vi "DynamicPersonality.vi"(7 "Pinned":T1={"Attacker"="Auto", "Striker"="Auto", "Defender"="Auto"}, 10 "our_goalie_id":dbl, 11 "input cluster":T3={"our_robots"=[], "enemy_robots"=[], "balls"=[], "geometry"={"line_width"=0, "field_length"=0, "field_width"=0, "boundary_width"=0, "referee_width"=0, "goal_width"=0, "goal_depth"=0, "goal_wall_width"=0, "center_circle_radius"=0, "defense_radius"=0, "defense_stretch"=0, "free_kick_from_defense_dist"=0, "penalty_spot_from_field_line_dist"=0, "penalty_line_from_spot_dist"=0}, "IA Judge"={"stage"="", "command"="", "our_goalie_id"=0.0, "enemy_goalie_id"=0.0, "command\nenum"=enum."Halt", "Time"=enum."Azul"}, "Received Timestamp"=timestamp(0 s since 1904-01-01), "Events"={"Touch"=FALSE, "Ball out"=FALSE, "id touch"=0.0, "Ball out of \nVision"=FALSE, "Ball inside \nGoalie area"=FALSE, "Robot not responding"=FALSE, "Robots responding status"=[1.0, 1.0, 1.0, 1.0, 1.0, 1.0], "Enemy Ball \nPossession"=FALSE}}) -> (2 "output cluster":T3={"our_robots"=[], "enemy_robots"=[], "balls"=[], "geometry"={"line_width"=0, "field_length"=0, "field_width"=0, "boundary_width"=0, "referee_width"=0, "goal_width"=0, "goal_depth"=0, "goal_wall_width"=0, "center_circle_radius"=0, "defense_radius"=0, "defense_stretch"=0, "free_kick_from_defense_dist"=0, "penalty_spot_from_field_line_dist"=0, "penalty_line_from_spot_dist"=0}, "IA Judge"={"stage"="", "command"="", "our_goalie_id"=0.0, "enemy_goalie_id"=0.0, "command\nenum"=enum."Halt", "Time"=enum."Azul"}, "Received Timestamp"=timestamp(0 s since 1904-01-01), "Events"={"Touch"=FALSE, "Ball out"=FALSE, "id touch"=0.0, "Ball out of \nVision"=FALSE, "Ball inside \nGoalie area"=FALSE, "Robot not responding"=FALSE, "Robots responding status"=[1.0, 1.0, 1.0, 1.0, 1.0, 1.0], "Enemy Ball \nPossession"=FALSE}})   [LabVIEW 2016]
uses:
  Core/AI Input.ctl
  Core/AI Robot.ctl
  Intel/Functions Enum.ctl
  Intel/AttackerStates.ctl
  Core/AI Ball.ctl
  Core/Field Size.ctl
  Core/AI Judge.ctl
  Intel/Command Enum.ctl
  Select Personalitys.ctl
  Util/Select Auto None or Robot.ctl
panel:
  out "Dfdr\nPinned?":bool
  in  "Qtd Min p/ Stk":dbl=5.0
  out "Strk\nPinned?":bool
  out "Attck\nPinned?":bool
  in  "Ids validos":u32[](array[numeric])=[42, 42, 42, 42, 42, 42, 42]
  out "Maior prioridade de \natacante é o mais\nproximo da bola?":bool
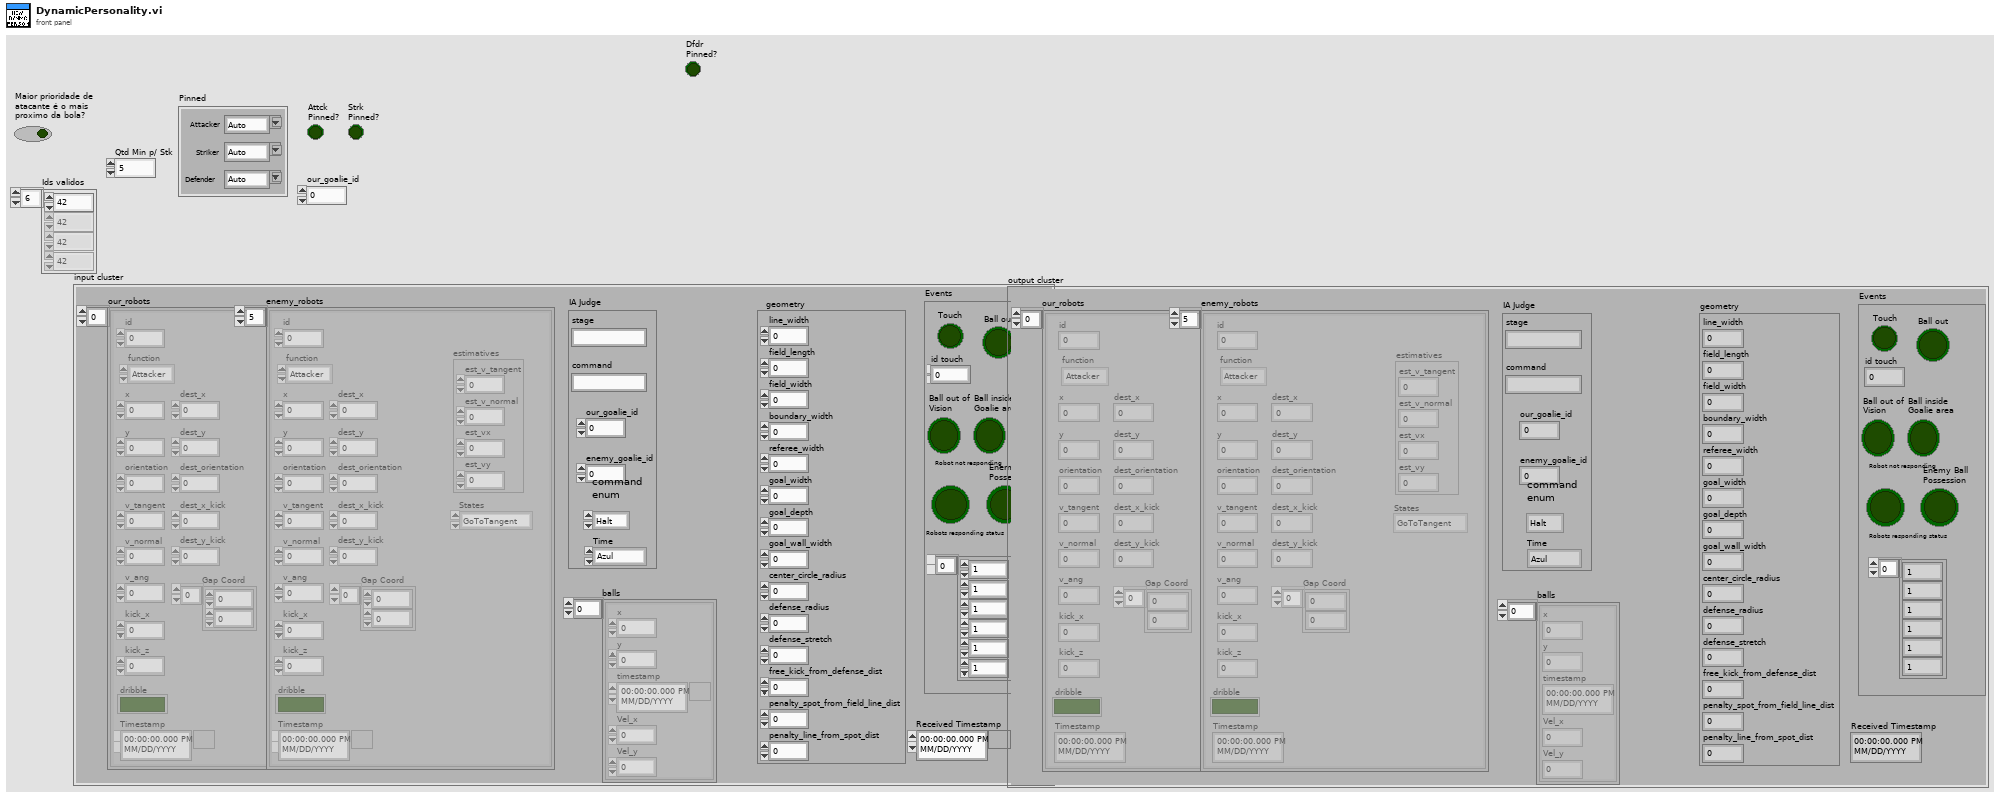
[diagram p1: front panel]
types:
  T1 = typedef "Select Personalitys.ctl" = cluster{"Attacker":T2, "Striker":T2, "Defender":T2}
  T2 = typedef "Select Auto None or Robot.ctl" = string
  T3 = typedef "AI Input.ctl" = cluster{"our_robots":T4[], "enemy_robots":T4[], "balls":T7[], "geometry":T8, "IA Judge":T9, "Received Timestamp":timestamp, "Events":cluster{"Touch":bool, "Ball out":bool, "id touch":dbl, "Ball out of \nVision":bool, "Ball inside \nGoalie area":bool, "Robot not responding":bool, "Robots responding status":dbl[], "Enemy Ball \nPossession":bool}}
  T4 = typedef "AI Robot.ctl" = cluster{"id":u32, "function":T5, "x":dbl, "y":dbl, "orientation":dbl, "v_tangent":dbl, "v_normal":dbl, "v_ang":dbl, "kick_x":dbl, "kick_z":dbl, "dribble":bool, "Timestamp":timestamp, "dest_x":dbl, "dest_y":dbl, "dest_orientation":dbl, "estimatives":cluster{"est_v_tangent":dbl, "est_v_normal":dbl, "est_vx":dbl, "est_vy":dbl}, "dest_x_kick":dbl, "dest_y_kick":dbl, "Gap Coord":dbl[], "States":T6}
  T5 = typedef "Functions Enum.ctl" = enum16{"Attacker", "Goalie", "Defender", "Striker", "Goto 0", "Dummy", "Kicker", "ZigZag"}
  T6 = typedef "AttackerStates.ctl" = enum16{"Pass", "GoToTangent", "BallGetting", "GoToKick", ""}
  T7 = typedef "AI Ball.ctl" = cluster{"x":dbl, "y":dbl, "timestamp":timestamp, "Vel_x":dbl, "Vel_y":dbl}
  T8 = typedef "Field Size.ctl" = cluster{"line_width":u32, "field_length":u32, "field_width":u32, "boundary_width":u32, "referee_width":u32, "goal_width":u32, "goal_depth":u32, "goal_wall_width":u32, "center_circle_radius":u32, "defense_radius":u32, "defense_stretch":u32, "free_kick_from_defense_dist":u32, "penalty_spot_from_field_line_dist":u32, "penalty_line_from_spot_dist":u32}
  T9 = typedef "AI Judge.ctl" = cluster{"stage":string, "command":string, "our_goalie_id":dbl, "enemy_goalie_id":dbl, "command\nenum":T10, "Time":enum16{"Azul", "Amarelo"}}
  T10 = typedef "Command Enum.ctl" = enum16{"Halt", "Stop", "Force Start", "PKA Normal Start", "Prepare Kickoff Ally", "PKE Normal Start", "Prepare Kickoff Enemy", "Prepare Penalty Ally", "PPA Normal Start", "Prepare Penalty Enemy", "PPE Normal Start", "Direct Free Enemy", "Direct Free Ally", "Indirect Free Enemy", "Indirect Free Ally", "Timeout Enemy", "Timeout Ally", "Goal Enemy", "Goal Ally", "Ball Placement Enemy", "Ball Placement Ally", "Normal Half Time", "Extra Time Break", "Extra Half Time", "None"}
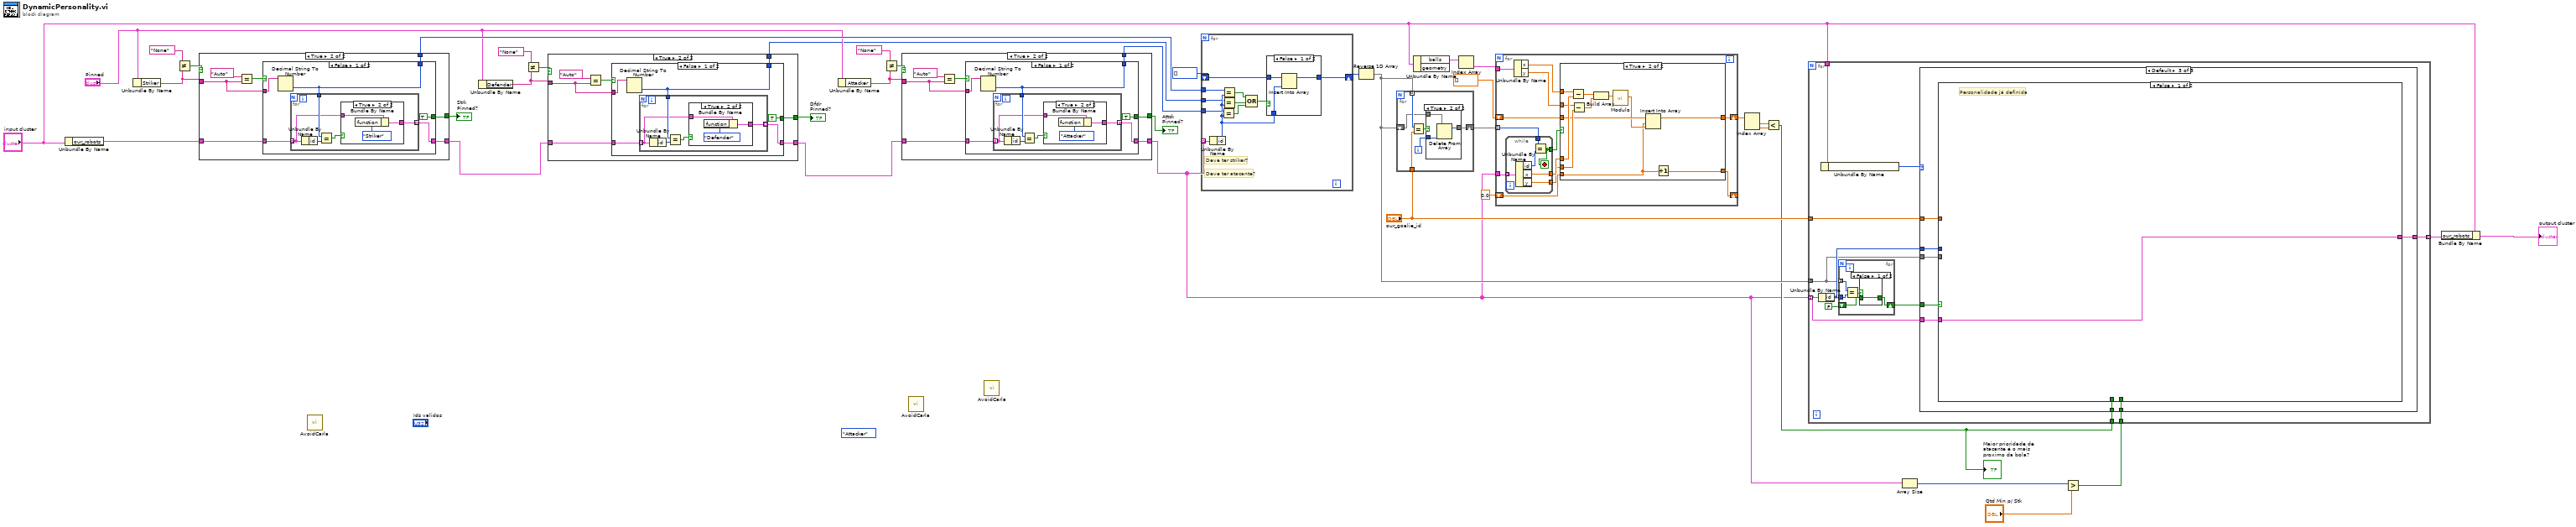
[diagram p0: block diagram]
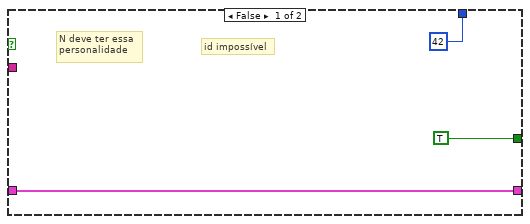
[diagram p2: hidden frame]
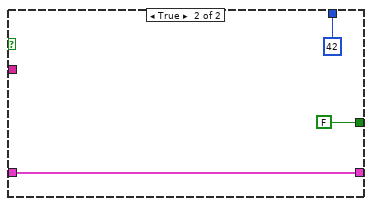
[diagram p4: hidden frame]
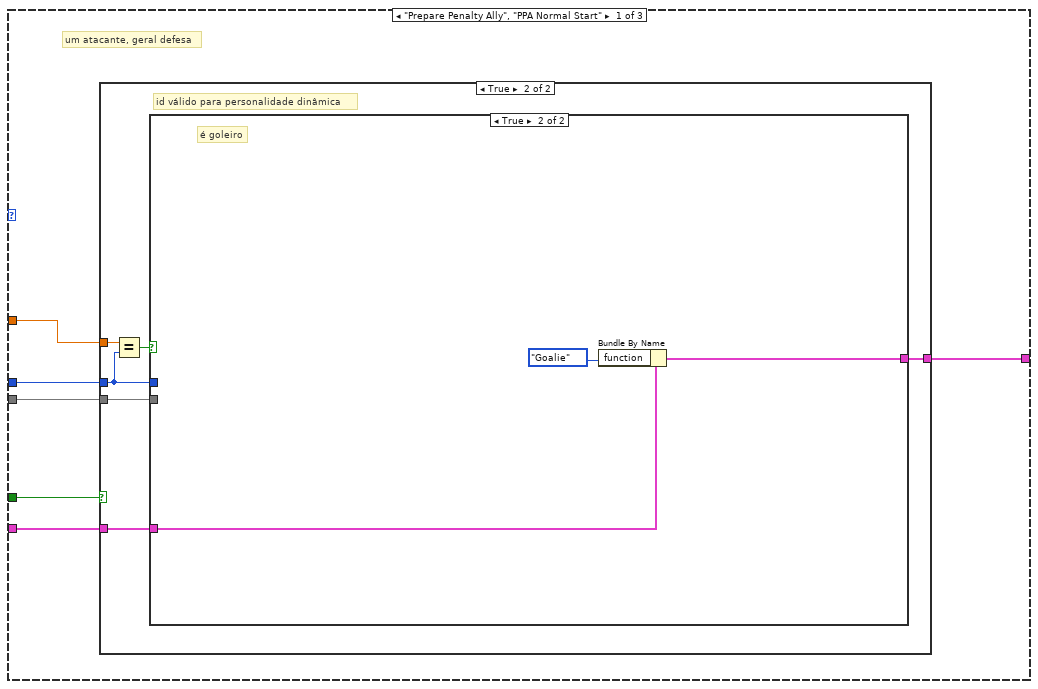
[diagram p7: hidden frame]
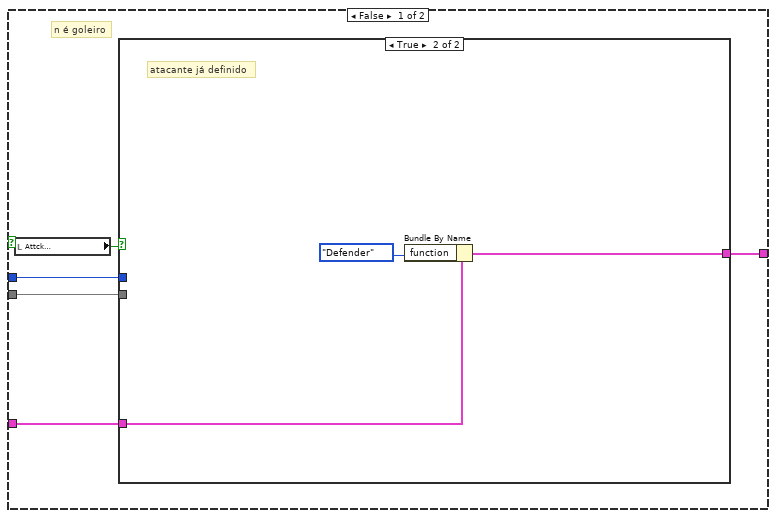
[diagram p9: hidden frame]
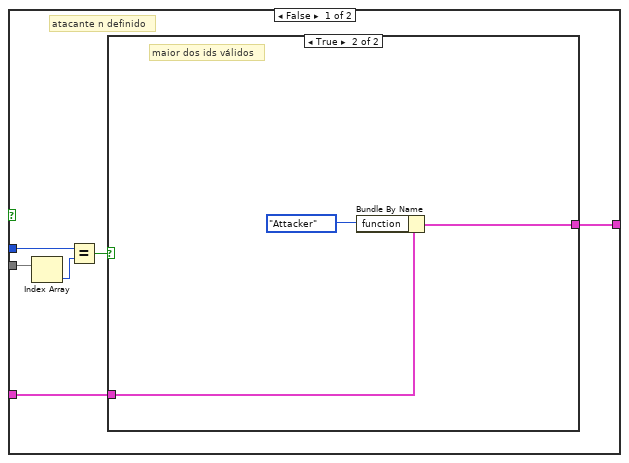
[diagram p10: hidden frame]
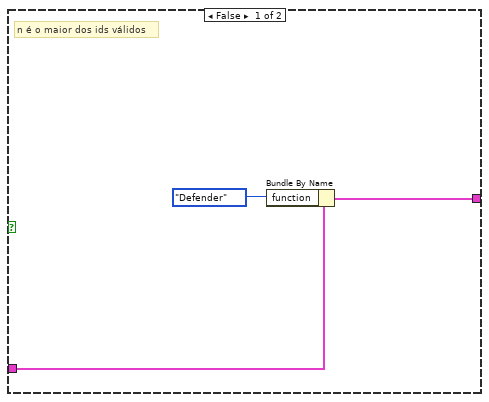
[diagram p11: hidden frame]
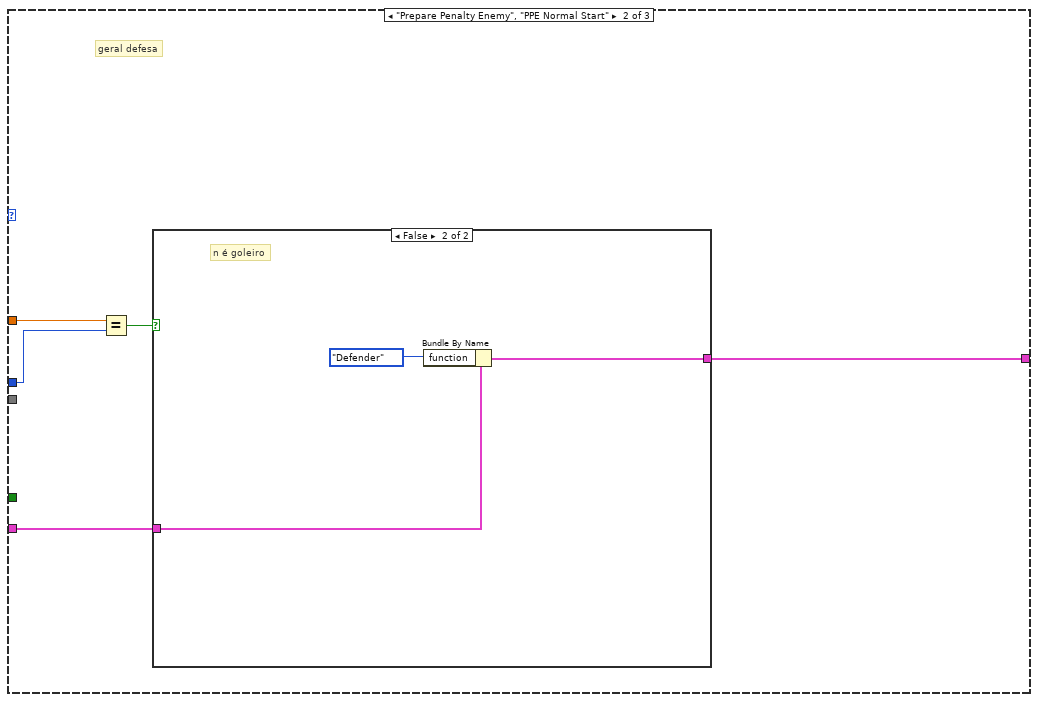
[diagram p12: hidden frame]
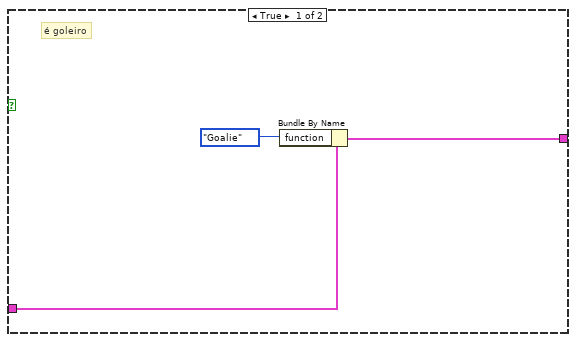
[diagram p13: hidden frame]
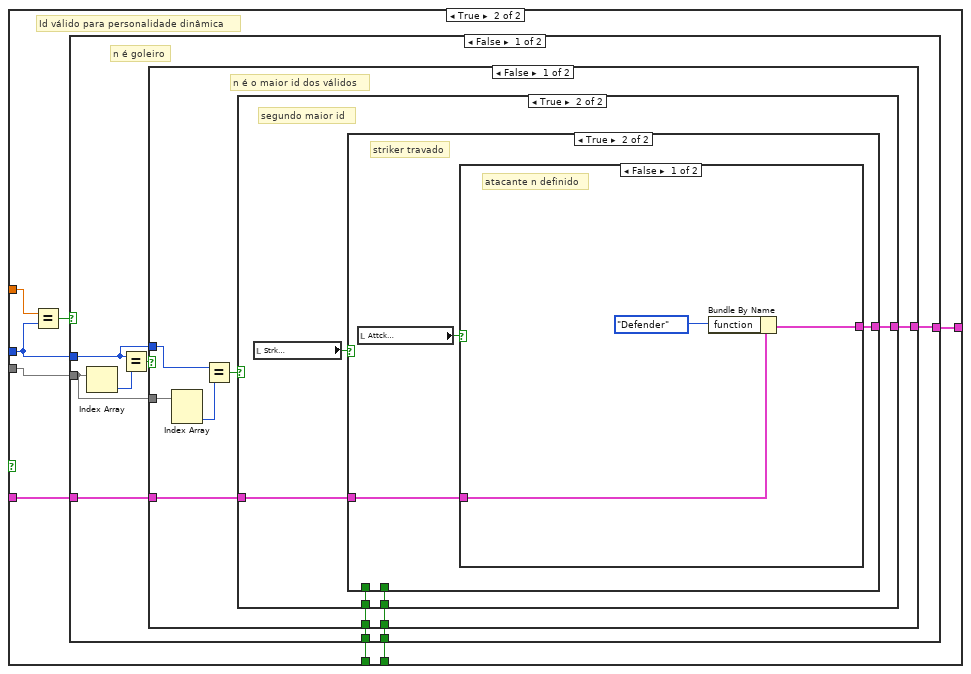
[diagram p14: hidden frame]
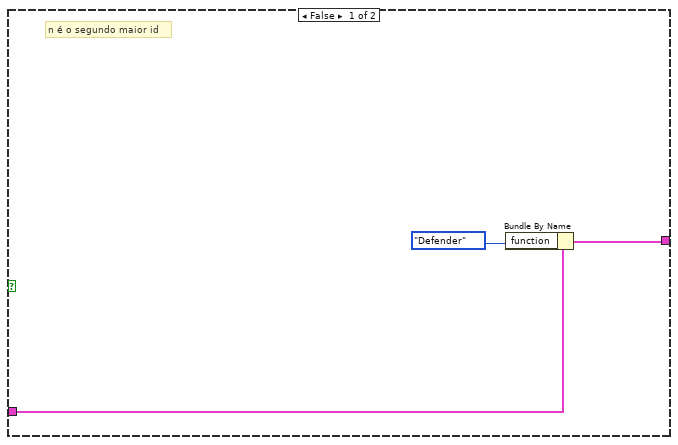
[diagram p15: hidden frame]
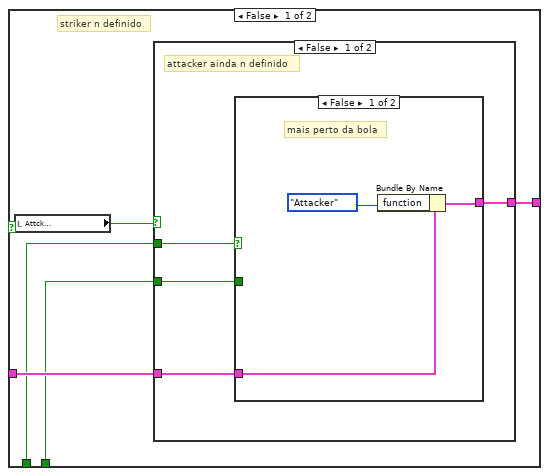
[diagram p16: hidden frame]
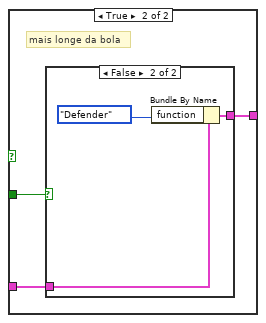
[diagram p17: hidden frame]
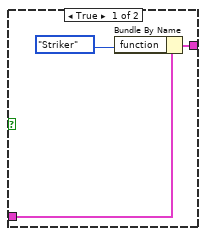
[diagram p18: hidden frame]
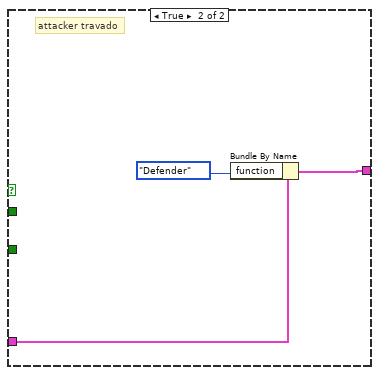
[diagram p19: hidden frame]
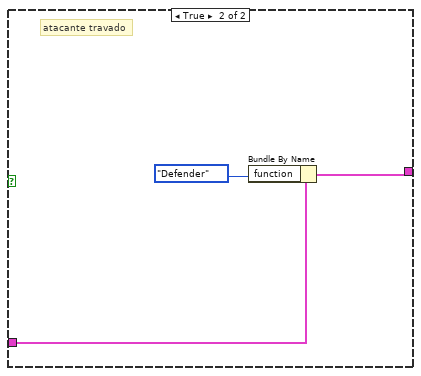
[diagram p20: hidden frame]
diagram:
  (unwired) Functions_Enum."Attacker" ("function")
  n1 = Unbundle By Name("input cluster") -> ("our_robots"=w36:T4[])
  n2 = Unbundle By Name("Pinned") -> ("Striker"=w37:T2)
  n3 = Not Equal?(x=T2 "None", y=w37) -> (x != y?=w38:bool)
  n4 = case shown="True" w38 {
    tunnel: w37 -> [_ w47]
    tunnel: w36 -> [w42 w46]
    tunnel: [w42 w45] -> w4
    tunnel: [TRUE w44] -> w10
    tunnel: [u32 42 ("Id Maior\nprioridade\natacante") w43] -> w31
    frame False {
      # "id impossível"
      # "N deve ter essa \npersonalidade"
    }
    frame True {
      n5 = Equal?(x=T2 "Auto", y=w47) -> (x = y?=w48:bool)
      n6 = case shown="False" w48 {
        tunnel: w47 -> [w54 _]
        tunnel: w46 -> [w53 w66]
        tunnel: [w52 w66] -> w45
        tunnel: [TRUE FALSE] -> w44
        tunnel: [w50 42] -> w43
        frame False {
          n7 = Decimal String To Number(string=w54) -> (number=w50:i32)  [unwired: 2 in, 1 out]
          n8 = for {
            tunnel: w53 -> [w57] mode=indexing
            tunnel: w50 -> [w58]
            tunnel: [w56] -> w52 mode=indexing
            n9 = Unbundle By Name(w57) -> ("id"=w59:u32)
            n10 = Equal?(x=w58, y=w59) -> (x = y?=w55:bool)
            n11 = case shown="True" w55 {
              tunnel: w57 -> [w60 w63]
              tunnel: [w60 w62] -> w56
              frame False {
              }
              frame True {
                n12 = Bundle By Name(cluster=w63, "function"=Functions_Enum."Striker") -> (w62:T4)
              }
            }
          }
        }
        frame True {
        }
      }
    }
  }
  "Strk\nPinned?" <- w10
  n13 = call "AvoidCarla.vi"() -> ()  [unwired: 11 in, 1 out]
  n14 = Unbundle By Name("Pinned") -> ("Defender"=w6:T2)
  n15 = Not Equal?(x=T2 "None", y=w6) -> (x != y?=w7:bool)
  n16 = case shown="True" w7 {
    tunnel: w6 -> [_ w74]
    tunnel: w4 -> [w69 w73]
    tunnel: [w69 w72] -> w3
    tunnel: [TRUE w71] -> w5
    tunnel: [u32 42 ("Id Maior\nprioridade\natacante") w70] -> w1
    frame False {
      # "id impossível"
      # "N deve ter essa \npersonalidade"
    }
    frame True {
      n17 = Equal?(x=T2 "Auto", y=w74) -> (x = y?=w75:bool)
      n18 = case shown="False" w75 {
        tunnel: w74 -> [w81 _]
        tunnel: w73 -> [w80 w93]
        tunnel: [w79 w93] -> w72
        tunnel: [TRUE FALSE] -> w71
        tunnel: [w77 42] -> w70
        frame False {
          n19 = Decimal String To Number(string=w81) -> (number=w77:i32)  [unwired: 2 in, 1 out]
          n20 = for {
            tunnel: w80 -> [w84] mode=indexing
            tunnel: w77 -> [w85]
            tunnel: [w83] -> w79 mode=indexing
            n21 = Unbundle By Name(w84) -> ("id"=w86:u32)
            n22 = Equal?(x=w85, y=w86) -> (x = y?=w82:bool)
            n23 = case shown="True" w82 {
              tunnel: w84 -> [w87 w90]
              tunnel: [w87 w89] -> w83
              frame False {
              }
              frame True {
                n24 = Bundle By Name(cluster=w90, "function"=Functions_Enum."Defender") -> (w89:T4)
              }
            }
          }
        }
        frame True {
        }
      }
    }
  }
  "Dfdr\nPinned?" <- w5
  n25 = Unbundle By Name("Pinned") -> ("Attacker"=w34:T2)
  n26 = Not Equal?(x=T2 "None", y=w34) -> (x != y?=w33:bool)
  n27 = case shown="True" w33 {
    tunnel: w34 -> [_ w101]
    tunnel: w3 -> [w96 w100]
    tunnel: [w96 w99] -> w13
    tunnel: [TRUE w98] -> w9
    tunnel: [42 w97] -> w32
    frame False {
      (unwired) u32 42 ("Id Maior\nprioridade\natacante")
      # "id impossível"
      # "N deve ter essa \npersonalidade"
    }
    frame True {
      n28 = Equal?(x=T2 "Auto", y=w101) -> (x = y?=w102:bool)
      n29 = case shown="False" w102 {
        tunnel: w101 -> [w108 _]
        tunnel: w100 -> [w107 w120]
        tunnel: [w106 w120] -> w99
        tunnel: [TRUE FALSE] -> w98
        tunnel: [w104 42] -> w97
        frame False {
          n30 = Decimal String To Number(string=w108) -> (number=w104:i32)  [unwired: 2 in, 1 out]
          n31 = for {
            tunnel: w107 -> [w111] mode=indexing
            tunnel: w104 -> [w112]
            tunnel: [w110] -> w106 mode=indexing
            n32 = Unbundle By Name(w111) -> ("id"=w113:u32)
            n33 = Equal?(x=w112, y=w113) -> (x = y?=w109:bool)
            n34 = case shown="True" w109 {
              tunnel: w111 -> [w114 w117]
              tunnel: [w114 w116] -> w110
              frame False {
              }
              frame True {
                n35 = Bundle By Name(cluster=w117, "function"=Functions_Enum."Attacker") -> (w116:T4)
              }
            }
          }
        }
        frame True {
        }
      }
    }
  }
  "Attck\nPinned?" <- w9
  n36 = call "AvoidCarla.vi"() -> ()  [unwired: 11 in, 1 out]
  n37 = call "AvoidCarla.vi"() -> ()  [unwired: 11 in, 1 out]
  n38 = for {
    tunnel: w13 -> [w131] mode=indexing
    tunnel: w32 -> [w130]
    shift-right: [w126] -> w29
    shift-left: u32[] [] -> [w127]
    tunnel: w31 -> [w129]
    tunnel: w1 -> [w123]
    # "Deve ter striker?"
    # "Deve ter atacante?"
    n39 = Unbundle By Name(w131) -> ("id"=w124:u32)
    n40 = Equal?(x=w130, y=w124) -> (x = y?=w128:bool)
    n41 = Equal?(x=w129, y=w124) -> (x = y?=w122:bool)
    n42 = Equal?(x=w123, y=w124) -> (x = y?=w121:bool)
    n43 = Compound Arithmetic op=OR(w122, w121, w128) -> (w125:bool)
    n44 = case shown="False" w125 {
      tunnel: [w132 w135] -> w126
      tunnel: w127 -> [w134 w135]
      tunnel: w124 -> [w133 _]
      frame False {
        n45 = Insert Into Array(array=w134, new element=w133) -> (w132:u32[])  [unwired: 1 in]
      }
      frame True {
      }
    }
  }
  n46 = Reverse 1D Array(array=w29) -> (reversed array=w25:u32[])
  n47 = for {
    tunnel: w25 -> [w140] mode=indexing
    tunnel: "our_goalie_id" -> [w139]
    shift-right: [w136] -> w22
    shift-left: w25 -> [w138]
    i -> [w137]
    n48 = Equal?(x=w140, y=w139) -> (x = y?=w141:bool)
    n49 = case shown="True" w141 {
      tunnel: w138 -> [w142 w145]
      tunnel: w137 -> [_ w144]
      tunnel: [w142 w143] -> w136
      frame False {
      }
      frame True {
        n50 = Delete From Array(array=w145, index=w144) -> (array with subset deleted=w143:u32[])  [unwired: 1 in, 1 out]
      }
    }
  }
  n51 = Unbundle By Name("input cluster") -> ("balls"=w24:T7[])  [unwired: 1 out]
  n52 = Index Array(array=w24) -> (element=w23:T7)  [unwired: 1 in]
  n53 = for {
    tunnel: w23 -> [w154]
    tunnel: w22 -> [w147] mode=indexing
    tunnel: w13 -> [w157]
    shift-right: [w151] -> w20
    shift-left: dbl[] [] -> [w150]
    shift-right: [w148] -> _
    shift-left: 0.0 -> [w149]
    n54 = while {
      tunnel: w157 -> [w163] mode=indexing
      tunnel: [w162] -> w156
      tunnel: [w161] -> w155
      tunnel: w147 -> [w160]
      tunnel: [w158] -> w146
      stop <- w158 stop-if-true
      n55 = Unbundle By Name(w163) -> ("id"=w159:u32, "x"=w162:dbl, "y"=w161:dbl)
      n56 = Equal?(x=w160, y=w159) -> (x = y?=w158:bool)
    }
    n57 = Unbundle By Name(w154) -> ("x"=w153:dbl, "y"=w152:dbl)
    n58 = case shown="True" w146 {
      tunnel: w156 -> [_ w176]
      tunnel: w155 -> [_ w174]
      tunnel: w153 -> [_ w177]
      tunnel: w152 -> [_ w175]
      tunnel: [w165 w170] -> w151
      tunnel: w150 -> [w165 w169]
      tunnel: w149 -> [w164 w167]
      tunnel: [w164 w166] -> w148
      frame False {
      }
      frame True {
        n59 = Subtract(x=w177, y=w176) -> (x-y=w173:dbl)
        n60 = Subtract(x=w175, y=w174) -> (x-y=w172:dbl)
        n61 = Build Array(w173, w172) -> (w171:dbl[])
        n62 = call "Modulo.vi"("2D vector"=w171) -> ("Modulo"=w168:dbl)  [unwired: 10 in]
        n63 = Insert Into Array(array=w169, index=w167, new element=w168) -> (w170:dbl[])
        n64 = Increment(x=w167) -> (x+1=w166:dbl)
      }
    }
  }
  n65 = Index Array(array=w20) -> (element #1=w18:dbl, element #2=w19:dbl)  [unwired: 2 in]
  n66 = Less?(x=w18, y=w19) -> (x < y?=w17:bool)
  "Maior prioridade de \natacante é o mais\nproximo da bola?" <- w17
  n67 = Array Size(array=w13) -> (size(s)=w12:i32)
  n68 = Greater?(x=w12, y="Qtd Min p/ Stk") -> (0:w15:bool)
  n69 = for {
    tunnel: w13 -> [w185] mode=indexing
    tunnel: w25 -> [w183]
    tunnel: "our_goalie_id" -> [w186]
    tunnel: [w184] -> w28 mode=indexing
    tunnel: w17 -> [w181]
    tunnel: w15 -> [w180]
    tunnel: "input cluster" -> [w179]
    n70 = Unbundle By Name(w185) -> ("id"=w187:u32)
    n71 = Unbundle By Name(w179) -> ("IA Judge.command\nenum"=w178:T10)
    n72 = for {
      tunnel: w183 -> [w360] mode=indexing
      tunnel: w187 -> [w361]
      shift-right: [w358] -> w182
      shift-left: FALSE -> [w359]
      n73 = Equal?(x=w360, y=w361) -> (x = y?=w357:bool)
      n74 = case shown="False" w357 {
        tunnel: w359 -> [w362 _]
        tunnel: [w362 TRUE] -> w358
        frame False {
        }
        frame True {
        }
      }
    }
    n75 = case shown="Default" w178 {
      tunnel: w187 -> [w191 w225 w243]
      tunnel: w186 -> [w189 w226 w242]
      tunnel: w185 -> [w193 w229 w241]
      tunnel: [w194 w228 w240] -> w184
      tunnel: w183 -> [w190 _ w239]
      tunnel: w182 -> [w192 _ w238]
      tunnel: w181 -> [_ _ w237]
      tunnel: w180 -> [_ _ w236]
      frame "Prepare Penalty Ally", "PPA Normal Start" {
        # "um atacante, geral defesa"
        n76 = case shown="True" w192 {
          tunnel: [w195 w201] -> w194
          tunnel: w193 -> [w195 w200]
          tunnel: w191 -> [_ w197]
          tunnel: w190 -> [_ w199]
          tunnel: w189 -> [_ w196]
          frame False {
            # "personalidade já definida"
          }
          frame True {
            # "id válido para personalidade dinâmica"
            n77 = Equal?(x=w196, y=w197) -> (x = y?=w198:bool)
            n78 = case shown="True" w198 {
              tunnel: [w206 w223] -> w201
              tunnel: w200 -> [w205 w222]
              tunnel: w197 -> [w203 _]
              tunnel: w199 -> [w202 _]
              frame False {
                # "n é goleiro"
                n79 = local read "Attck\nPinned?"() -> (w204:bool)
                n80 = case shown="True" w204 {
                  tunnel: [w212 w220] -> w206
                  tunnel: w205 -> [w211 w219]
                  tunnel: w203 -> [w209 _]
                  tunnel: w202 -> [w207 _]
                  frame False {
                    # "atacante n definido"
                    n81 = Index Array(array=w207) -> (element=w208:u32)  [unwired: 1 in]
                    n82 = Equal?(x=w209, y=w208) -> (x = y?=w210:bool)
                    n83 = case shown="True" w210 {
                      tunnel: [w214 w217] -> w212
                      tunnel: w211 -> [w213 w216]
                      frame False {
                        # "n é o maior dos ids válidos"
                        n84 = Bundle By Name(cluster=w213, "function"=Functions_Enum."Defender") -> (w214:T4)
                      }
                      frame True {
                        # "maior dos ids válidos"
                        n85 = Bundle By Name(cluster=w216, "function"=Functions_Enum."Attacker") -> (w217:T4)
                      }
                    }
                  }
                  frame True {
                    # "atacante já definido"
                    n86 = Bundle By Name(cluster=w219, "function"=Functions_Enum."Defender") -> (w220:T4)
                  }
                }
              }
              frame True {
                # "é goleiro"
                n87 = Bundle By Name(cluster=w222, "function"=Functions_Enum."Goalie") -> (w223:T4)
              }
            }
          }
        }
      }
      frame "Prepare Penalty Enemy", "PPE Normal Start" {
        # "geral defesa"
        n88 = Equal?(x=w226, y=w225) -> (x = y?=w227:bool)
        n89 = case shown="False" w227 {
          tunnel: w229 -> [w232 w235]
          tunnel: [w231 w234] -> w228
          frame True {
            # "é goleiro"
            n90 = Bundle By Name(cluster=w232, "function"=Functions_Enum."Goalie") -> (w231:T4)
          }
          frame False {
            # "n é goleiro"
            n91 = Bundle By Name(cluster=w235, "function"=Functions_Enum."Defender") -> (w234:T4)
          }
        }
      }
      frame Default {
        n92 = case shown="False" w238 {
          tunnel: w243 -> [_ w248]
          tunnel: w242 -> [_ w252]
          tunnel: w241 -> [w244 w250]
          tunnel: [w244 w249] -> w240
          tunnel: w239 -> [_ w247]
          tunnel: w237 -> [_ w246]
          tunnel: w236 -> [_ w245]
          frame False {
            # "Personalidade já definida"
          }
          frame True {
            # "Id válido para personalidade dinâmica"
            n93 = Equal?(x=w252, y=w248) -> (x = y?=w251:bool)
            n94 = case shown="False" w251 {
              tunnel: w250 -> [w257 w355]
              tunnel: [w258 w354] -> w249
              tunnel: w248 -> [w255 _]
              tunnel: w247 -> [w256 _]
              tunnel: w246 -> [w254 _]
              tunnel: w245 -> [w253 _]
              frame False {
                # "n é goleiro"
                n95 = Index Array(array=w256) -> (element=w259:u32)  [unwired: 1 in]
                n96 = Equal?(x=w255, y=w259) -> (x = y?=w260:bool)
                n97 = case shown="False" w260 {
                  tunnel: [w265 w313] -> w258
                  tunnel: w257 -> [w266 w312]
                  tunnel: w256 -> [w267 _]
                  tunnel: w255 -> [w264 _]
                  tunnel: w254 -> [w262 w311]
                  tunnel: w253 -> [w261 w310]
                  frame False {
                    # "n é o maior id dos válidos"
                    n98 = Index Array(array=w267) -> (element #2=w263:u32)  [unwired: 2 in, 1 out]
                    n99 = Equal?(x=w264, y=w263) -> (x = y?=w268:bool)
                    n100 = case shown="True" w268 {
                      tunnel: w266 -> [w269 w275]
                      tunnel: [w270 w274] -> w265
                      tunnel: w262 -> [_ w273]
                      tunnel: w261 -> [_ w272]
                      frame False {
                        # "n é o segundo maior id"
                        n101 = Bundle By Name(cluster=w269, "function"=Functions_Enum."Defender") -> (w270:T4)
                      }
                      frame True {
                        # "segundo maior id"
                        n102 = local read "Strk\nPinned?"() -> (w276:bool)
                        n103 = case shown="True" w276 {
                          tunnel: w275 -> [w280 w302]
                          tunnel: [w281 w301] -> w274
                          tunnel: w273 -> [w278 _]
                          tunnel: w272 -> [w277 _]
                          frame False {
                            # "striker n definido"
                            n104 = local read "Attck\nPinned?"() -> (w279:bool)
                            n105 = case shown="False" w279 {
                              tunnel: [w285 w299] -> w281
                              tunnel: w280 -> [w284 w298]
                              tunnel: w278 -> [w283 _]
                              tunnel: w277 -> [w282 _]
                              frame False {
                                # "attacker ainda n definido"
                                n106 = case shown="False" w283 {
                                tunnel: [w287 w291] -> w285
                                tunnel: w284 -> [w286 w290]
                                tunnel: w282 -> [_ w289]
                                frame False {
                                # "mais perto da bola"
                                n107 = Bundle By Name(cluster=w286, "function"=Functions_Enum."Attacker") -> (w287:T4)
                                }
                                frame True {
                                # "mais longe da bola"
                                n108 = case shown="False" w289 {
                                tunnel: [w293 w296] -> w291
                                tunnel: w290 -> [w292 w295]
                                frame True {
                                n109 = Bundle By Name(cluster=w292, "function"=Functions_Enum."Striker") -> (w293:T4)
                                }
                                frame False {
                                n110 = Bundle By Name(cluster=w295, "function"=Functions_Enum."Defender") -> (w296:T4)
                                }
                                }
                                }
                                }
                              }
                              frame True {
                                # "attacker travado"
                                n111 = Bundle By Name(cluster=w298, "function"=Functions_Enum."Defender") -> (w299:T4)
                              }
                            }
                          }
                          frame True {
                            # "striker travado"
                            n112 = local read "Attck\nPinned?"() -> (w303:bool)
                            n113 = case shown="False" w303 {
                              tunnel: w302 -> [w304 w307]
                              tunnel: [w305 w308] -> w301
                              frame False {
                                # "atacante n definido"
                                n114 = Bundle By Name(cluster=w304, "function"=Functions_Enum."Defender") -> (w305:T4)
                              }
                              frame True {
                                # "atacante travado"
                                n115 = Bundle By Name(cluster=w307, "function"=Functions_Enum."Defender") -> (w308:T4)
                              }
                            }
                          }
                        }
                      }
                    }
                  }
                  frame True {
                    # "maior id dos válidos"
                    n116 = local read "Attck\nPinned?"() -> (w314:bool)
                    n117 = case shown="True" w314 {
                      tunnel: [w318 w340] -> w313
                      tunnel: w312 -> [w317 w339]
                      tunnel: w311 -> [w316 _]
                      tunnel: w310 -> [w315 w338]
                      frame False {
                        # "Atacante ainda n definido"
                        n118 = case shown="True" w316 {
                          tunnel: [w322 w336] -> w318
                          tunnel: w317 -> [w321 w335]
                          tunnel: w315 -> [w319 _]
                          frame False {
                            # "n é o mais perto da bola"
                            n119 = local read "Strk\nPinned?"() -> (w320:bool)
                            n120 = case shown="False" w320 {
                              tunnel: [w325 w333] -> w322
                              tunnel: w321 -> [w324 w332]
                              tunnel: w319 -> [w323 _]
                              frame False {
                                n121 = case shown="False" w323 {
                                tunnel: [w327 w330] -> w325
                                tunnel: w324 -> [w326 w329]
                                frame True {
                                n122 = Bundle By Name(cluster=w326, "function"=Functions_Enum."Striker") -> (w327:T4)
                                }
                                frame False {
                                n123 = Bundle By Name(cluster=w329, "function"=Functions_Enum."Defender") -> (w330:T4)
                                }
                                }
                              }
                              frame True {
                                n124 = Bundle By Name(cluster=w332, "function"=Functions_Enum."Attacker") -> (w333:T4)
                              }
                            }
                          }
                          frame True {
                            # "mais perto da bola"
                            n125 = Bundle By Name(cluster=w335, "function"=Functions_Enum."Attacker") -> (w336:T4)
                          }
                        }
                      }
                      frame True {
                        # "Atacande já travado"
                        n126 = local read "Strk\nPinned?"() -> (w341:bool)
                        n127 = case shown="True" w341 {
                          tunnel: [w344 w352] -> w340
                          tunnel: w339 -> [w343 w351]
                          tunnel: w338 -> [w342 _]
                          frame False {
                            # "Striker ainda n definido"
                            n128 = case shown="False" w342 {
                              tunnel: [w346 w349] -> w344
                              tunnel: w343 -> [w345 w348]
                              frame True {
                                n129 = Bundle By Name(cluster=w345, "function"=Functions_Enum."Striker") -> (w346:T4)
                              }
                              frame False {
                                n130 = Bundle By Name(cluster=w348, "function"=Functions_Enum."Defender") -> (w349:T4)
                              }
                            }
                          }
                          frame True {
                            # "Sobra defesa"
                            # "Striker já travado"
                            n131 = Bundle By Name(cluster=w351, "function"=Functions_Enum."Defender") -> (w352:T4)
                          }
                        }
                      }
                    }
                  }
                }
              }
              frame True {
                # "é goleiro"
                n132 = Bundle By Name(cluster=w355, "function"=Functions_Enum."Goalie") -> (w354:T4)
              }
            }
          }
        }
      }
    }
  }
  n133 = Bundle By Name(cluster="input cluster", "our_robots"=w28) -> (→"output cluster":T3)
